vi "IZRCSM_ut_test.vi"(8 "Error In":errorcluster, 11 "CSMinfo in":T3) -> (0 "Error Out":errorcluster, 3 "CSMinfo out":T3)   [LabVIEW 2018]
uses:
  MOKO_LabViewLibrary/MokoSTM/MokoClassicUtilitySTM/MCUS_ITEM.ctl
  MOKO_LabViewLibrary/MokoSTM/MokoClassicUtilitySTM/MCUS_STM.ctl
  IZRCSM.ctl
  IZRCSM_string.ctl
  IZRCSM_string2.ctl
panel:
  in  "Применить":bool
  in  "Температура окружающего воздуха":T1
  in  "Атмосферное давление":T1
  in  "Относительная влажность воздуха":T1
  in  "Дата завершения испытаний":T2
  in  "Дата начала испытаний":T2
  in  "Методы испытаний (измерений)":T2
  in  "НД, устанавливающий требования":T2
  in  "IMEI образца":T2
  in  "Идентификация (шифр) образца":T2
  in  "Регистрационный номер заказа":T2
  # "1. Общие сведения"
  # "Регистрационный номер заказа:"
  # "0,4\n0,6\n1\n1,5\n1,6\n2,5\n4"
  # "kPa\nbar\nkgf/cm2\nMPa"
  # "Идентификация (шифр) образца:"
  # "IMEI образца:"
  # "НД, устанавливающий требования:"
  # "Методы испытаний (измерений):"
  # "Дата начала испытаний:"
  # "Дата завершения испытаний:"
  # "2. Климатические условия внешней среды"
  # "Допустимый диапазон по \n ГОСТ 33470-2015 (п.6.2.4)"
  # "Измеренные значения"
  # "Измеряемый параметр"
  # "Температура окружающего воздуха:"
  # "от +15,0 °C до +35,0 °C"
  # "Относительная влажность воздуха:"
  # "от 45% до 80%"
  # "Атмосферное давление:"
  # "от 84,0 до 106,7 кПа"
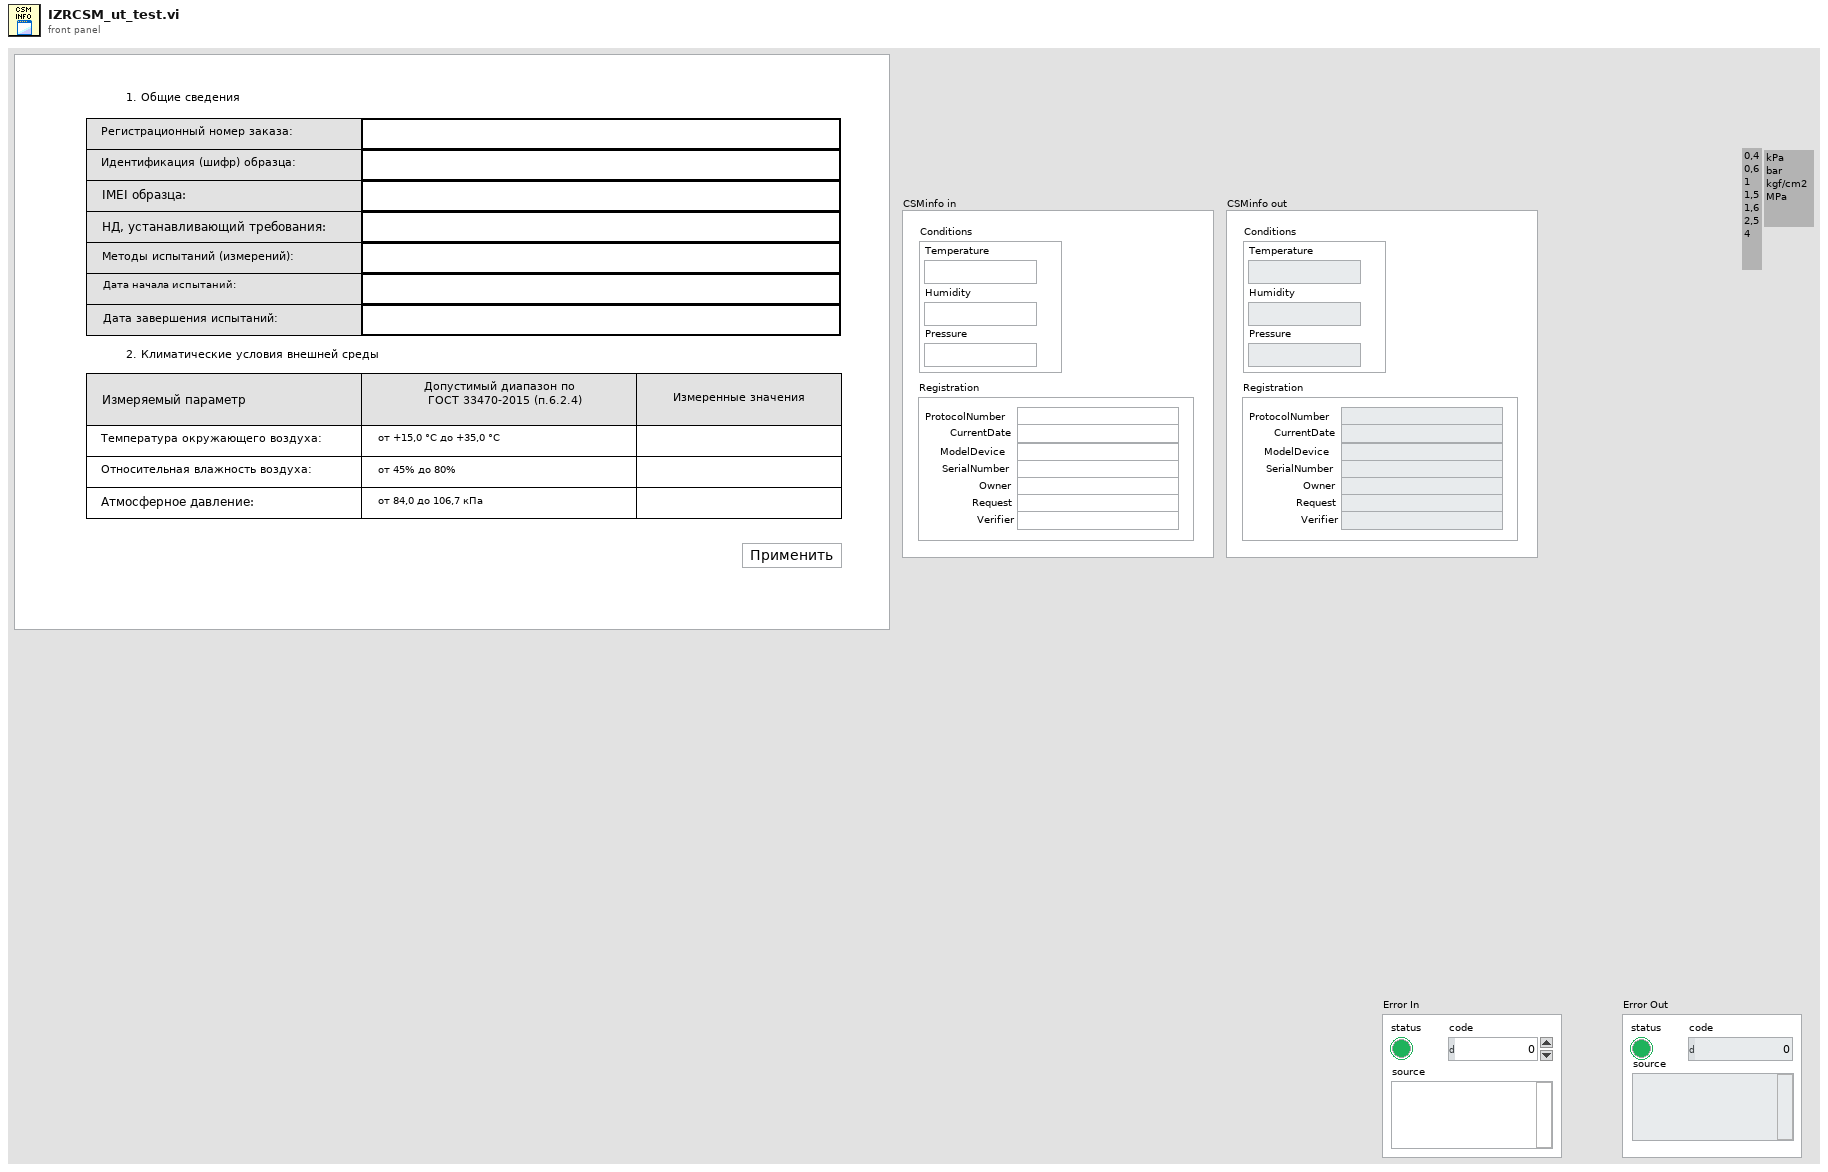
[diagram p1: front panel]
types:
  T1 = typedef "IZRCSM_string2.ctl" = string
  T2 = typedef "IZRCSM_string.ctl" = string
  T3 = typedef "IZRCSM.ctl" = cluster{"Conditions":cluster{"Temperature":string, "Humidity":string, "Pressure":string}, "Registration":cluster{"ProtocolNumber":string, "CurrentDate":string, "ModelDevice":string, "SerialNumber":string, "Owner":string, "Request":string, "Verifier":string}}
  T4 = typedef "MCUS_STM.ctl" = cluster{"main stm":T5, "data":string}
  T5 = typedef "MCUS_ITEM.ctl" = enum16{"idle", "_____ main_____ ", "Init", "Stop", "Apply values", "Save", "Open", "Reset"}
  T6 = cluster{"Регистрационный номер заказа":string, "Идентификация (шифр) образца":string, "IMEI образца":string, "НД, устанавливающий требования":string, "Методы испытаний (измерений)":string, "Дата начала испытаний":string, "Дата завершения испытаний":string}
  T7 = cluster{"Температура окружающего воздуха":string, "Относительная влажность воздуха":string, "Атмосферное давление":string}
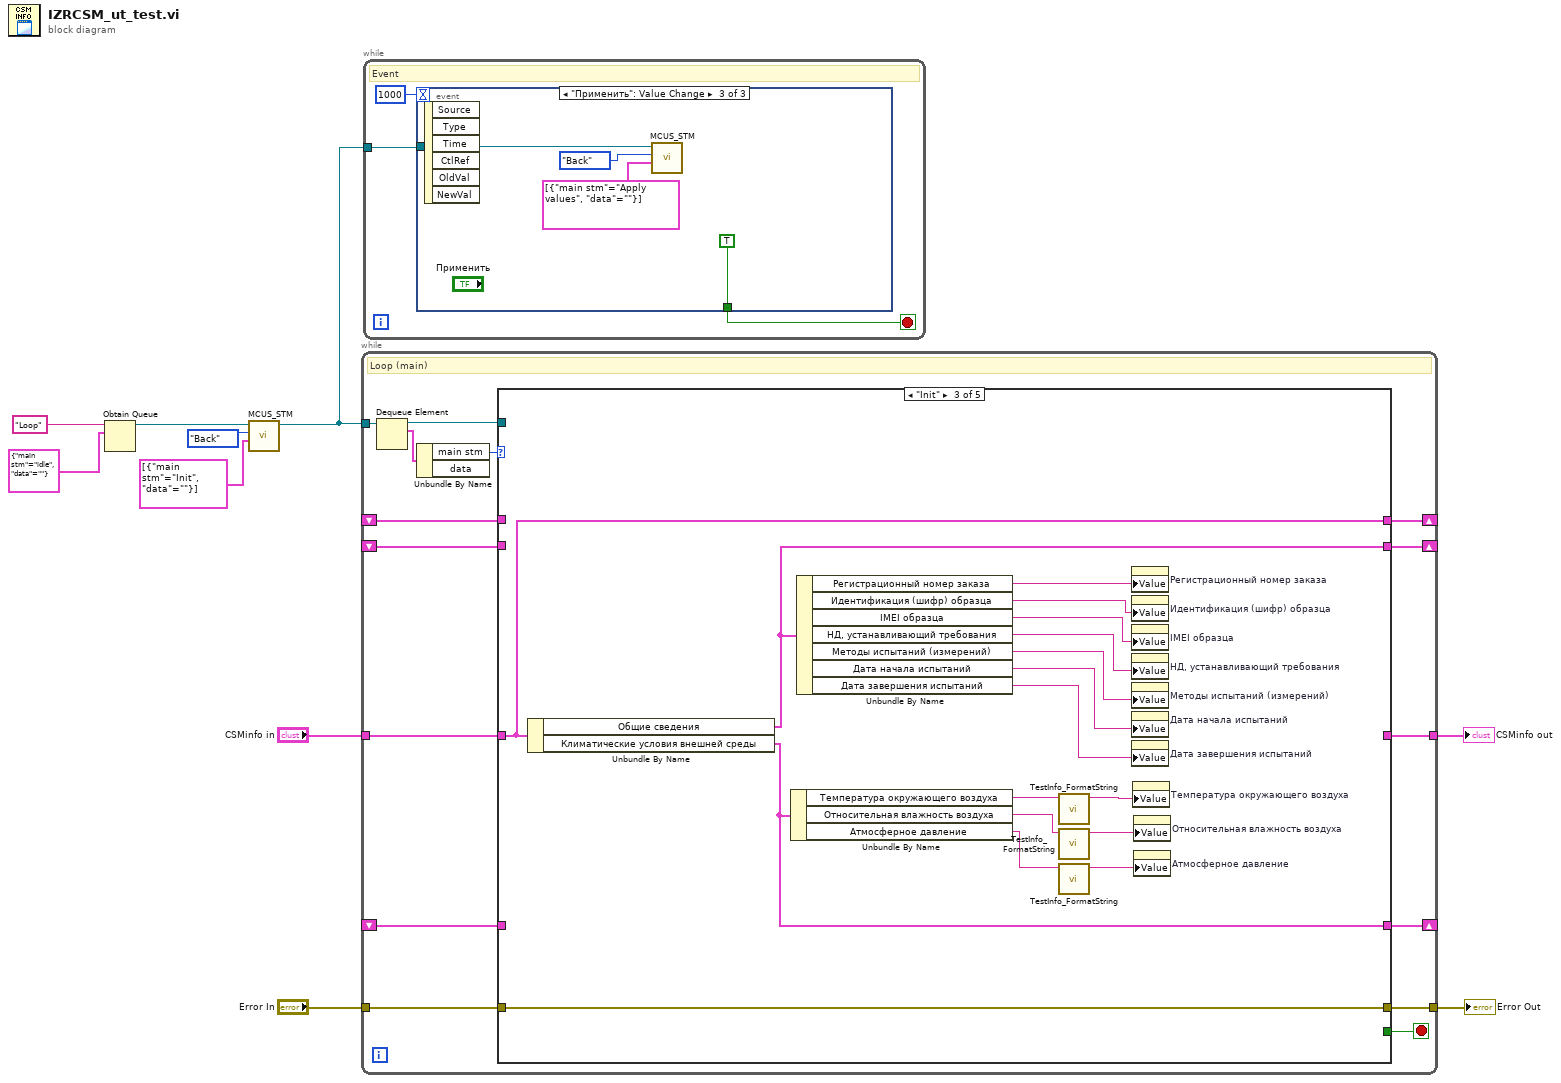
[diagram p0: block diagram]
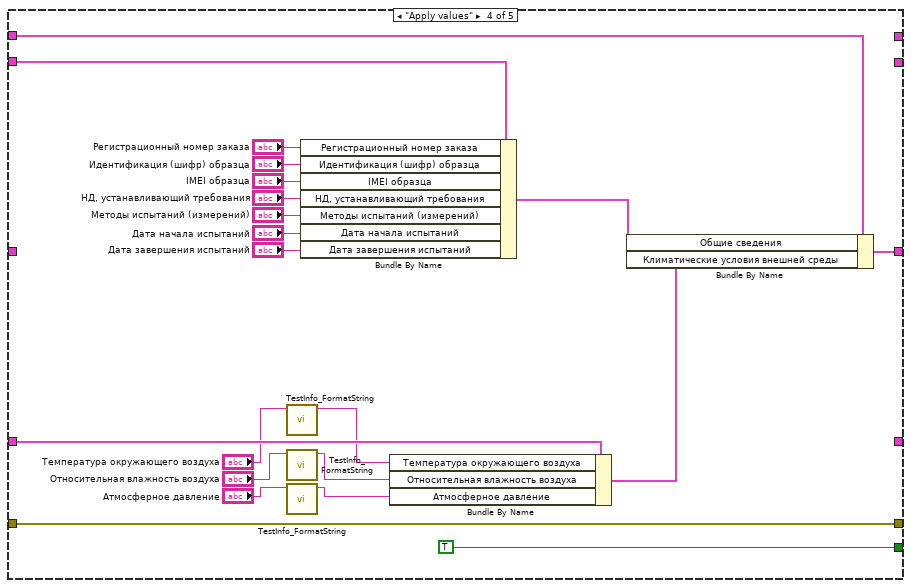
[diagram p4: hidden frame]
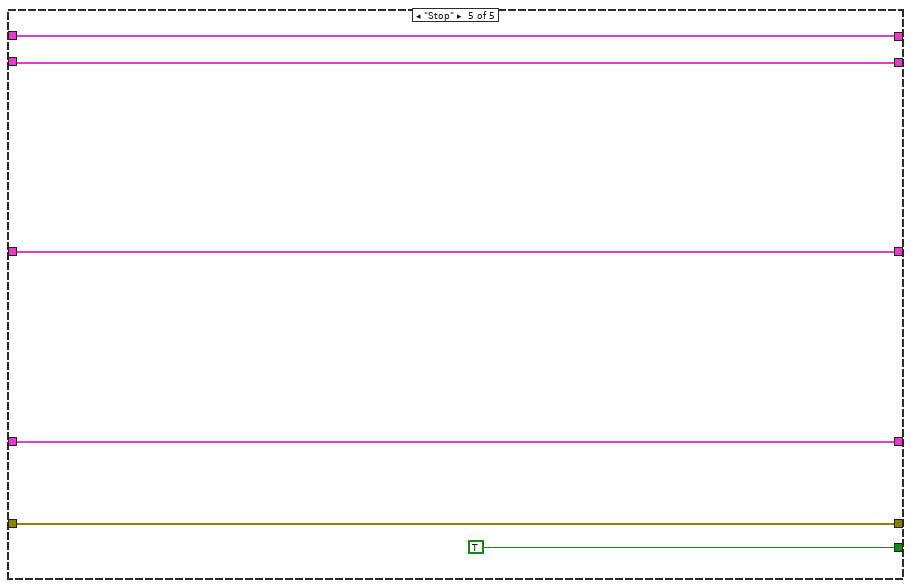
[diagram p5: hidden frame]
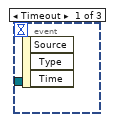
[diagram p6: hidden frame]
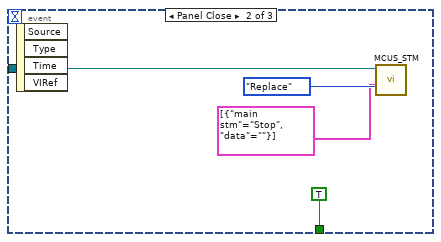
[diagram p7: hidden frame]
diagram:
  n1 = Obtain Queue(name (unnamed)="Loop", element data type=T4 {"main stm"=enum."idle", "data"=""} ("MOKO_NMEA")) -> (queue out=w10:refnum<queue>)  [unwired: 3 in, 2 out]
  n2 = call "MCUS_STM.vi"("StateMachineSteps"=T4[] [{"main stm"=enum."Init", "data"=""}], "FNs"=enum16{"Back", "Front", "Replace"}."Back", "Queue in"=w10) -> ("Queue out"=w5:refnum<queue>)  [unwired: 7 in, 1 out]
  n3 = while {
    tunnel: w5 -> [w25]
    shift-right: [w21] -> _
    shift-left: _ -> [w13]
    shift-right: [w20] -> _
    shift-left: _ -> [w14]
    tunnel: [w18] -> w4
    tunnel: "CSMinfo in" -> [w17]
    tunnel: "Error In" -> [w16]
    tunnel: [w15] -> w1
    shift-right: [w12] -> _
    shift-left: _ -> [w11]
    stop <- w19 stop-if-true
    # "Loop (main)"
    n4 = Dequeue Element(queue=w25) -> (queue out=w24:refnum<queue>, element=w23:T4)  [unwired: 2 in, 2 out]
    n5 = Unbundle By Name(w23) -> ("main stm"=w22:T5)  [unwired: 1 out]
    n6 = case shown="\"Init\"" w22 {
      tunnel: w24 -> [_ _ _ _ _]
      tunnel: [w27 _ w44 _ w68] -> w21
      tunnel: w14 -> [w28 _ _ w61 w69]
      tunnel: [w28 _ w36 _ w69] -> w20
      tunnel: w13 -> [w27 _ _ w62 w68]
      tunnel: [_ _ _ TRUE TRUE] -> w19
      tunnel: [_ _ _ w65 w71] -> w18
      tunnel: w17 -> [_ _ w36 _ w71]
      tunnel: w16 -> [_ _ w45 w64 w70]
      tunnel: [_ _ w45 w64 w70] -> w15
      tunnel: [w26 _ w35 _ w67] -> w12
      tunnel: w11 -> [w26 _ _ w60 w67]
      frame "idle", Default {
      }
      frame "_____ main_____ " {
      }
      frame "Init" {
        n7 = Unbundle By Name(w36) -> ("Общие сведения"=w44:T6, "Климатические условия внешней среды"=w35:T7)
        n8 = Unbundle By Name(w35) -> ("Температура окружающего воздуха"=w32:string, "Относительная влажность воздуха"=w30:string, "Атмосферное давление"=w34:string)
        n9 = Unbundle By Name(w44) -> ("Регистрационный номер заказа"=w43:string, "Идентификация (шифр) образца"=w42:string, "IMEI образца"=w41:string, "НД, устанавливающий требования"=w40:string, "Методы испытаний (измерений)"=w39:string, "Дата начала испытаний"=w38:string, "Дата завершения испытаний"=w37:string)
        n10 = call "TestInfo_FormatString.vi"("Input string"=w32) -> ("resulting string"=w31:string)  [unwired: 9 in, 1 out]
        n11 = call "TestInfo_FormatString.vi"("Input string"=w30) -> ("resulting string"=w29:string)  [unwired: 9 in, 1 out]
        n12 = call "TestInfo_FormatString.vi"("Input string"=w34) -> ("resulting string"=w33:string)  [unwired: 9 in, 1 out]
        n13 = property on="Регистрационный номер заказа" class="Str (strict)"("Value"=w43) -> ()  [unwired: 2 in, 2 out]
        n14 = property on="Идентификация (шифр) образца" class="Str (strict)"("Value"=w42) -> ()  [unwired: 2 in, 2 out]
        n15 = property on="IMEI образца" class="Str (strict)"("Value"=w41) -> ()  [unwired: 2 in, 2 out]
        n16 = property on="НД, устанавливающий требования" class="Str (strict)"("Value"=w40) -> ()  [unwired: 2 in, 2 out]
        n17 = property on="Методы испытаний (измерений)" class="Str (strict)"("Value"=w39) -> ()  [unwired: 2 in, 2 out]
        n18 = property on="Дата начала испытаний" class="Str (strict)"("Value"=w38) -> ()  [unwired: 2 in, 2 out]
        n19 = property on="Дата завершения испытаний" class="Str (strict)"("Value"=w37) -> ()  [unwired: 2 in, 2 out]
        n20 = property on="Температура окружающего воздуха" class="Str (strict)"("Value"=w31) -> ()  [unwired: 2 in, 2 out]
        n21 = property on="Относительная влажность воздуха" class="Str (strict)"("Value"=w29) -> ()  [unwired: 2 in, 2 out]
        n22 = property on="Атмосферное давление" class="Str (strict)"("Value"=w33) -> ()  [unwired: 2 in, 2 out]
      }
      frame "Apply values" {
        n23 = call "TestInfo_FormatString.vi"("Input string"="Температура окружающего воздуха") -> ("resulting string"=w46:string)  [unwired: 9 in, 1 out]
        n24 = call "TestInfo_FormatString.vi"("Input string"="Относительная влажность воздуха") -> ("resulting string"=w47:string)  [unwired: 9 in, 1 out]
        n25 = call "TestInfo_FormatString.vi"("Input string"="Атмосферное давление") -> ("resulting string"=w48:string)  [unwired: 9 in, 1 out]
        n26 = Bundle By Name(cluster=w62, "Регистрационный номер заказа"="Регистрационный номер заказа", "Идентификация (шифр) образца"="Идентификация (шифр) образца", "IMEI образца"="IMEI образца", "НД, устанавливающий требования"="НД, устанавливающий требования", "Методы испытаний (измерений)"="Методы испытаний (измерений)", "Дата начала испытаний"="Дата начала испытаний", "Дата завершения испытаний"="Дата завершения испытаний") -> (w63:T6)
        n27 = Bundle By Name(cluster=w60, "Температура окружающего воздуха"=w46, "Относительная влажность воздуха"=w47, "Атмосферное давление"=w48) -> (w59:T7)
        n28 = Bundle By Name(cluster=w61, "Общие сведения"=w63, "Климатические условия внешней среды"=w59) -> (w65:T3)
      }
      frame "Stop" {
      }
    }
  }
  "CSMinfo out" <- w4
  "Error Out" <- w1
  n29 = while {
    tunnel: w5 -> [w73]
    stop <- w75 stop-if-true
    # "Event"
    n30 = event shown="[2] \"Применить\": Value Change" {
      selector: _ -> [_ _ _]
      dyn-events: _ -> [_ _ _]
      timeout: 1000 -> [_ _ _]
      tunnel: [_ TRUE TRUE] -> w75
      tunnel: w73 -> [_ w76 w81]
      event Timeout {
        n31 = event-data() -> ()  [unwired: 1 in, 3 out]
      }
      event Panel Close {
        n32 = event-data() -> ()  [unwired: 1 in, 4 out]
        n33 = call "MCUS_STM.vi"("StateMachineSteps"=T4[] [{"main stm"=enum."Stop", "data"=""}], "FNs"=enum16{"Back", "Front", "Replace"}."Replace", "Queue in"=w76) -> ()  [unwired: 7 in, 2 out]
      }
      event "Применить": Value Change {
        n34 = event-data() -> ()  [unwired: 1 in, 6 out]
        n35 = call "MCUS_STM.vi"("StateMachineSteps"=T4[] [{"main stm"=enum."Apply values", "data"=""}], "FNs"=enum16{"Back", "Front", "Replace"}."Back", "Queue in"=w81) -> ()  [unwired: 7 in, 2 out]
      }
    }
  }
